vi "Pockels Cal-Update cal file.vi"(8 "error in (no error)":errorcluster, 9 "Cal files listbox":refnum<vi>, 10 "New cal section":string[][](array[string])) -> (0 "error out":errorcluster)   [LabVIEW 2013]
uses:
  Typedefs/Which path.ctl
  Program Files (x86)/National Instruments/LabVIEW 2013/user.lib/My Palettes.lib/Files & paths/Spreadsheet/Read From Spreadsheet File (string)-Mod.vi
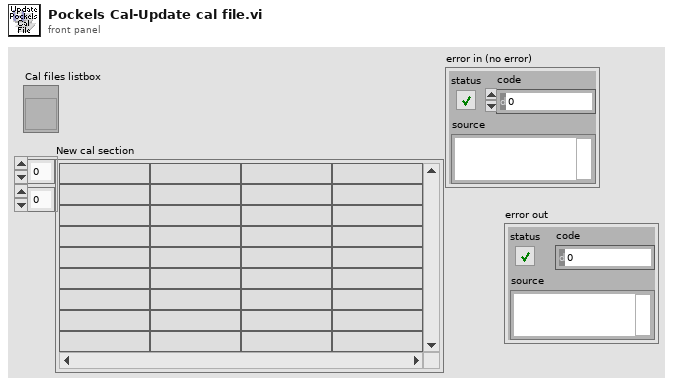
[diagram p1: front panel]
types:
  T1 = typedef "Which path.ctl" = enum16{"Configuration Files", "Calibration Files", "Images", "Setup.ini", "Loaded User profile.ini", "User's-Previous session.ini", "New user profile.ini", "Selected User profile.ini", "User profiles folder", "Power meter scaling.txt", "FOV Cal.ini"}
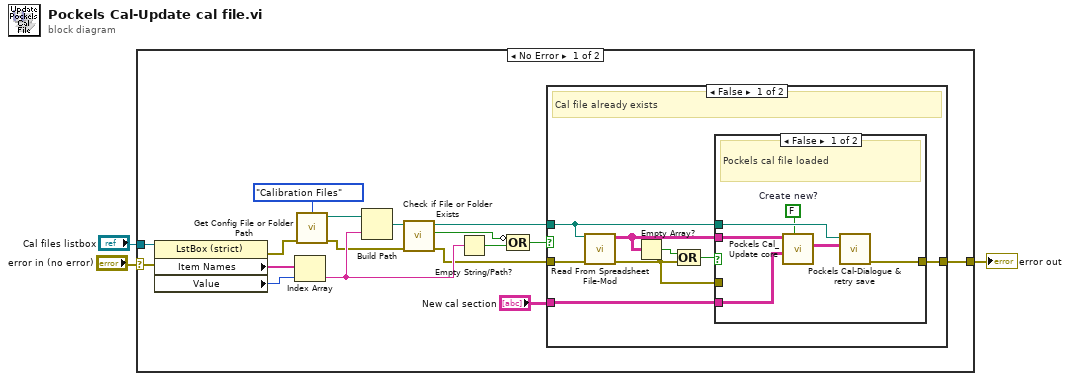
[diagram p0: block diagram]
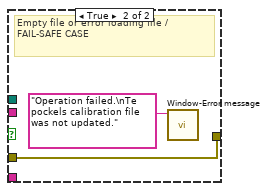
[diagram p2: hidden frame]
diagram:
  n1 = case shown="No Error" "error in (no error)" {
    selector: "error in (no error)" -> [w4 w38]
    tunnel: "Cal files listbox" -> [w12 _]
    tunnel: [w8 w38] -> w1
    frame No Error {
      n2 = property on="Property Node" class="LstBox (strict)"(reference=w12, error in=w4) -> (error out=w5:errorcluster, "Item Names"=w11:string[], "Value"=w10:i32)  [unwired: 1 out]
      n3 = Index Array(array=w11, index=w10) -> (element=w9:string)
      n4 = call "Get Config File or Folder Path.vi"("Error In"=w5, "Which file or folder?"=Which_path."Calibration Files" ("Which path?")) -> ("Error Out"=w6:errorcluster, "File Path"=w19:path)  [unwired: 7 in, 1 out]
      n5 = Build Path(base path=w19, name or relative path=w9) -> (appended path=w17:path)
      n6 = call <vilib>:"Check if File or Folder Exists.vi"("error in (no error)"=w6, "path"=w17) -> ("error out"=w7:errorcluster, "file or folder exists?"=w15:bool, "dup path"=w16:path)  [unwired: 7 in]
      n7 = Empty String/Path?(string/path=w9) -> (empty?=w14:bool)
      n8 = Compound Arithmetic op=OR(invert w15, w14) -> (w13:bool)
      n9 = case shown="False" w13 {
        tunnel: "New cal section" -> [w24 _]
        tunnel: w16 -> [w25 _]
        tunnel: [w23 w37] -> w8
        tunnel: w7 -> [w22 w37]
        frame False {
          # "Cal file already exists"
          n10 = call-poly "Read From Spreadsheet File-Mod.vi"("file path (dialog if empty)"=w25, "error in"=w22) -> ("all rows"=w26:string[][], "error out"=w21:errorcluster)  [unwired: 8 in, 4 out]
          n11 = Empty Array?(array=w26) -> (empty?=w28:bool)
          n12 = Compound Arithmetic op=OR(w28, w21) -> (w27:bool)
          n13 = case shown="False" w27 {
            tunnel: w24 -> [w34 _]
            tunnel: w26 -> [w33 _]
            tunnel: w25 -> [w31 _]
            tunnel: [w30 w35] -> w23
            tunnel: w21 -> [_ w35]
            frame False {
              w29 = FALSE  # Create new?
              # "Pockels cal file loaded"
              n14 = call "Pockels Cal_Update core.vi"("Create new?"=w29, "New cal section (empty objectives removed)"=w34, "Loaded cal file"=w33) -> ("Cal file strings"=w32:string[][])  [unwired: 8 in]
              n15 = call "Pockels Cal-Dialogue & retry save.vi"("Pockels Cal table"=w32, "Pockels cal file path"=w31) -> ("error out"=w30:errorcluster)  [unwired: 9 in]
            }
            frame True {
              # "Empty file or error loading file / FAIL-SAFE CASE"
              n16 = call "Window-Error message.vi"("Message"="Operation failed.\nTe pockels calibration file was not updated.") -> ()  [unwired: 10 in, 1 out]
            }
          }
        }
        frame True {
          # "Cal file not found or cal file name is empty"
        }
      }
    }
    frame Error {
    }
  }
  "error out" <- w1
